vi "Line Sensor AE.vi"(0 "AE State":T2) -> (1 "Line Detected?":bool, 2 "Line Sensor Raw Values":T1)   [LabVIEW 2018]
uses:
  Line Sensor AE Type Def.ctl
  <vilib>/myRIO/Common/Instrument Driver Framework/myRIO v1.0/AI/typedefs/AI Channels List.ctl
  <vilib>/myRIO/Common/Instrument Driver Framework/myRIO v1.0/AI/typedefs/AI Channels Enum.ctl
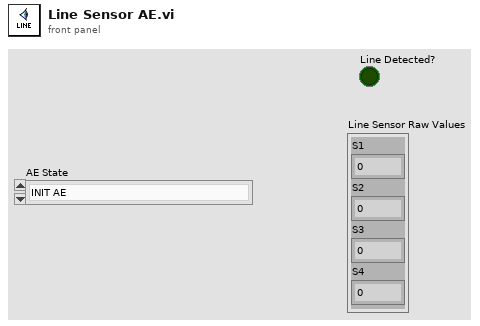
[diagram p1: front panel]
types:
  T1 = cluster{"S1":dbl, "S2":dbl, "S3":dbl, "S4":dbl, "Array[4]":dbl, "Array[5]":dbl, "Array[6]":dbl, "Array[7]":dbl, "Array[8]":dbl}
  T2 = typedef "Line Sensor AE Type Def.ctl" = enum16{"INIT AE", "READ FROM LINE SENSORS"}
  T3 = cluster{"Array[0]":dbl, "Array[1]":dbl, "Array[2]":dbl, "Array[3]":dbl, "Array[4]":dbl, "Array[5]":dbl, "Array[6]":dbl, "Array[7]":dbl, "Array[8]":dbl}
  T4 = typedef "AI Channels List.ctl" = T5[]
  T5 = typedef "AI Channels Enum.ctl" = enum16{"Not Connected", "AudioIn/Left", "AudioIn/Right", "C/AI0", "C/AI1", "A/AI0", "A/AI1", "A/AI2", "A/AI3", "A/AI4", "A/AI5", "A/AI6", "A/AI7", "B/AI0", "B/AI1", "B/AI2", "B/AI3", "B/AI4", "B/AI5", "B/AI6", "B/AI7", "AI/AI0", "AI/AI1", "AI/AI2", "AI/AI3", "A/AI0 (DIFF)", "A/AI1 (DIFF)", "A/AI2 (DIFF)", "A/AI3 (DIFF)", "B/AI0 (DIFF)", "B/AI1 (DIFF)", "B/AI2 (DIFF)", "B/AI3 (DIFF)"}
  T6 = typedef "Analog Scaling Constants List.ctl" = T7[]
  T7 = typedef "Analog Scaling Constants.ctl" = cluster{"LSB Weight (Volts)":dbl, "Offset (Volts)":dbl, "Signed?":bool}
  T8 = cluster{"Scale Constants Array":T6, "FPGA Reference Out":refnum<k20>, "AI Channel":T4}
  T9 = cluster{"Array[0]":bool, "Array[1]":bool, "Array[2]":bool, "Array[3]":bool, "Array[4]":bool, "Array[5]":bool, "Array[6]":bool, "Array[7]":bool, "Array[8]":bool}
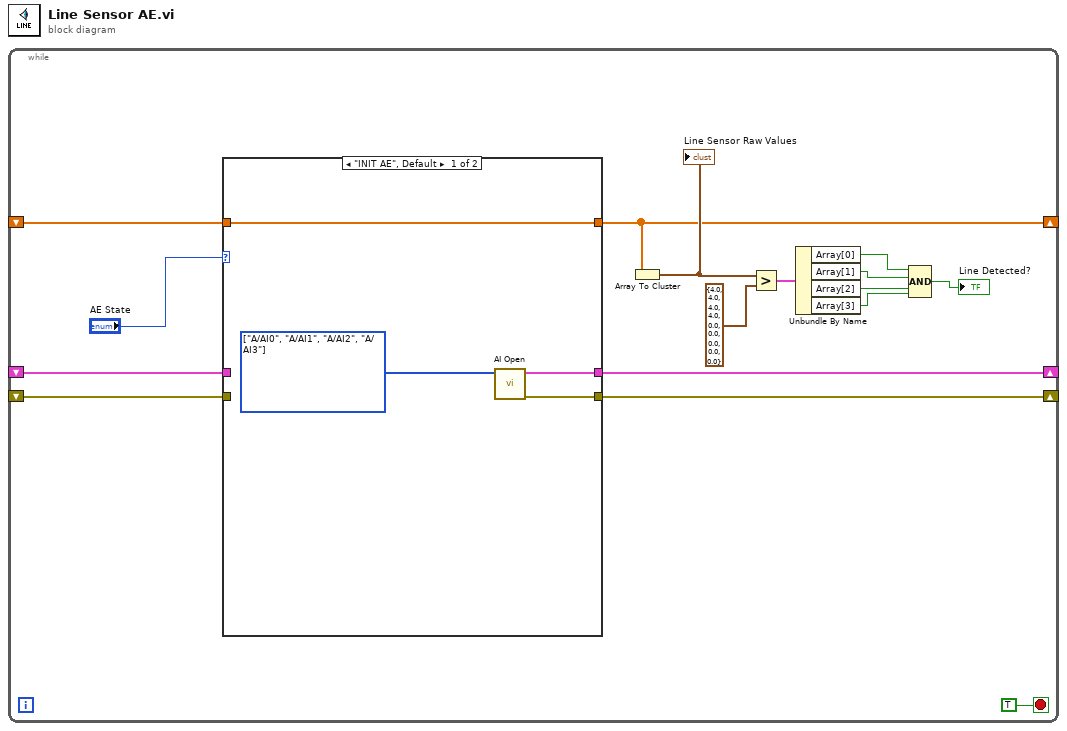
[diagram p0: block diagram]
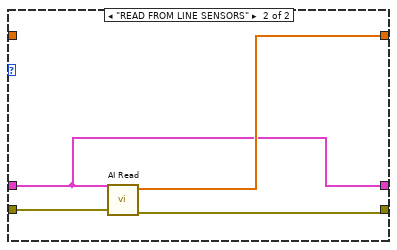
[diagram p2: hidden frame]
diagram:
  n1 = while {
    shift-right: [w15] -> _
    shift-left: _ -> [w13]
    shift-right: [w14] -> _
    shift-left: _ -> [w12]
    shift-right: [w2] -> _
    shift-left: _ -> [w1]
    stop <- TRUE stop-if-true
    n2 = case shown="\"INIT AE\", Default" "AE State" {
      tunnel: [w20 w21] -> w15
      tunnel: [w18 w23] -> w14
      tunnel: w13 -> [_ w21]
      tunnel: w12 -> [_ w24]
      tunnel: [w17 w22] -> w2
      tunnel: w1 -> [w17 _]
      frame "INIT AE", Default {
        w19 = T4 [enum."A/AI0", enum."A/AI1", enum."A/AI2", enum."A/AI3"] items=["Not Connected", "AudioIn/Left", "AudioIn/Right", "C/AI0", "C/AI1", "A/AI0", "A/AI1", "A/AI2", "A/AI3", "A/AI4", "A/AI5", "A/AI6", "A/AI7", "B/AI0", "B/AI1", "B/AI2", "B/AI3", "B/AI4", "B/AI5", "B/AI6", "B/AI7", "AI/AI0", "AI/AI1", "AI/AI2", "AI/AI3", "A/AI0 (DIFF)", "A/AI1 (DIFF)", "A/AI2 (DIFF)", "A/AI3 (DIFF)", "B/AI0 (DIFF)", "B/AI1 (DIFF)", "B/AI2 (DIFF)", "B/AI3 (DIFF)"] ("AI Channel")
        n3 = call <vilib>:"AI Open.vi"("AI Channel"=w19) -> ("error out"=w18:errorcluster, "Analog Info"=w20:T8)  [unwired: 9 in]
      }
      frame "READ FROM LINE SENSORS" {
        n4 = call <vilib>:"AI Read.vi"("error in (no error)"=w24, "Analog Info"=w21) -> ("error out"=w23:errorcluster, "Array"=w22:dbl[])  [unwired: 8 in]
      }
    }
    n5 = Array To Cluster(array=w2) -> (cluster=w11:T3)
    "Line Sensor Raw Values" <- w11
    n6 = Greater?(x=w11, y=T3 {"Array[0]"=4.0, "Array[1]"=4.0, "Array[2]"=4.0, "Array[3]"=4.0, "Array[4]"=0.0, "Array[5]"=0.0, "Array[6]"=0.0, "Array[7]"=0.0, "Array[8]"=0.0}) -> (0:w9:T9)
    n7 = Unbundle By Name(w9) -> ("Array[0]"=w8:bool, "Array[1]"=w7:bool, "Array[2]"=w6:bool, "Array[3]"=w5:bool)
    n8 = Compound Arithmetic op=AND(w8, w7, w6, w5) -> (→"Line Detected?":bool)
  }
